vi "create.addOrderLong.vi"(11 "AddOrder.Parms":T1={"Time Offset"=447000, "Order Id"="ORID0001", "Side Indicator"="B", "Quantity"=20000, "Symbol"="AAPL", "Price"=0.905, "Add Flags"=1}) -> (2 "Bytes.Out":u8[](array[numeric])=[34, 33, 24, 210, 6, 0, 79, 82, 73, 68, 48, 48, 48, 49, 66, 32, 78, 0, 0, 65, 65, 80, 76, 32, 32, 90, 35, 0, 0, 0, 0, 0, 0, 1] format="%.0x", 3 "AddOrderLong out":refnum<class "AddOrderLong.lvclass">)   [LabVIEW 2022 SP3]
uses:
  AddOrderLong/AddOrderLong.lvclass
  AddOrderLong/AddOrderLong.Parameters.ctl
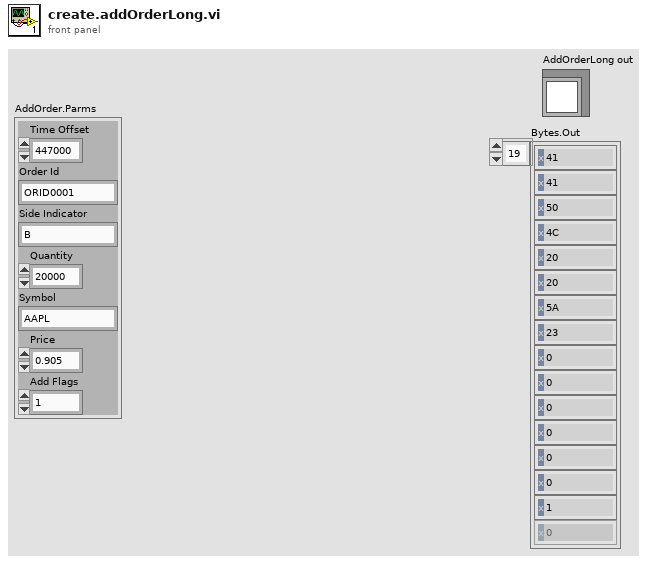
[diagram p1: front panel]
types:
  T1 = typedef "AddOrderLong.lvclass/AddOrderLong.Parameters.ctl" = cluster{"Time Offset":u32, "Order Id":string, "Side Indicator":string, "Quantity":u32, "Symbol":string, "Price":dbl, "Add Flags":u8}
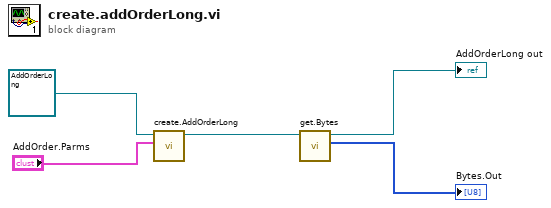
[diagram p0: block diagram]
diagram:
  n1 = call "create.AddOrderLong.vi"("AddOrder.Parms"="AddOrder.Parms", "AddOrderLong in"=refnum<class "AddOrderLong.lvclass"> refnum ("AddOrderLong.lvclass")) -> ("AddOrderLong out"=w4:refnum<class "AddOrderLong.lvclass">)  [unwired: 8 in, 1 out]
  n2 = call-dynamic "get.Bytes.vi"("PitchMessage in"=w4) -> ("Bytes.Out"=→"Bytes.Out":u8[], "PitchMessage out"=→"AddOrderLong out":refnum<class "AddOrderLong.lvclass">)  [unwired: 8 in, 1 out]
